vi "Format Wavename.vi"(8 "error in (no error)":errorcluster, 9 "Index":i32, 10 "Path":path, 11 "Name":string) -> (0 "error out":errorcluster, 3 "Formatted wavename":string)   [LabVIEW 2016, in "LV-Data.ITX.lvclass"]
uses:
  LV-Data.ITX.lvclass
  LV-Data/LV-Data.lvclass
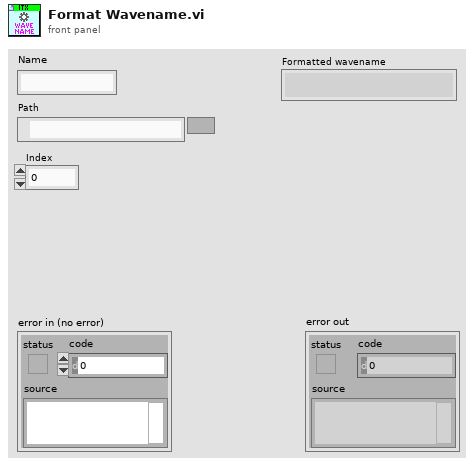
[diagram p1: front panel]
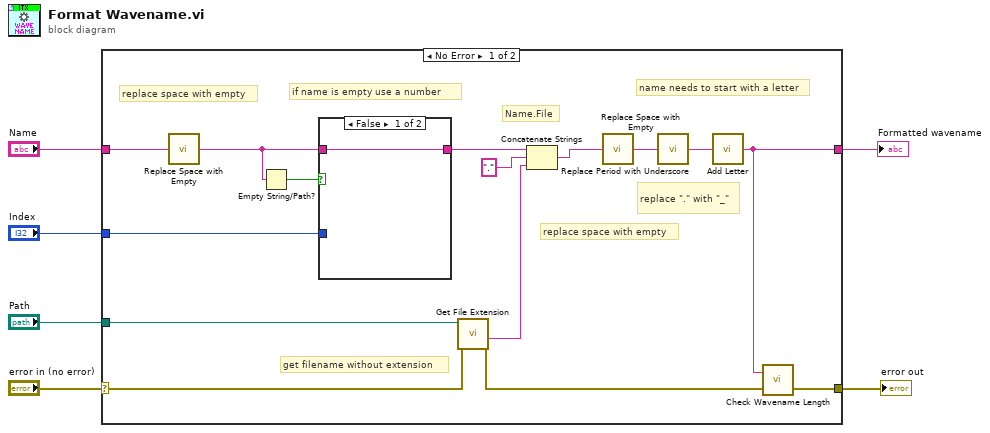
[diagram p0: block diagram]
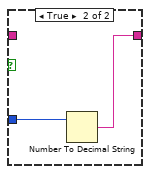
[diagram p2: hidden frame]
diagram:
  n1 = case shown="No Error" "error in (no error)" {
    selector: "error in (no error)" -> [w14 w26]
    tunnel: "Name" -> [w21 w25]
    tunnel: "Index" -> [w18 _]
    tunnel: "Path" -> [w16 _]
    tunnel: [w10 w25] -> w1
    tunnel: [w12 w26] -> w3
    frame No Error {
      # "replace space with empty"
      # "name needs to start with a letter"
      # "Name.File"
      # "if name is empty use a number"
      # "get filename without extension"
      # "replace \".\" with \"_\""
      # "replace space with empty"
      n2 = call "Replace Space with Empty.vi"("string"=w21) -> ("result string"=w13:string)
      n3 = Empty String/Path?(string/path=w13) -> (empty?=w17:bool)
      n4 = case shown="False" w17 {
        tunnel: w18 -> [_ w23]
        tunnel: [w22 w24] -> w19
        tunnel: w13 -> [w22 _]
        frame False {
        }
        frame True {
          n5 = Number To Decimal String(number=w23) -> (decimal integer string=w24:string)  [unwired: 1 out]
        }
      }
      n6 = call <vilib>:"Get File Extension.vi"("error in (no error)"=w14, "file"=w16) -> ("error out"=w9:errorcluster, "filename without extension"=w15:string)  [unwired: 5 in, 3 out]
      n7 = Concatenate Strings(w19, "." ("string"), w15) -> (w8:string)
      n8 = call "Replace Space with Empty.vi"("string"=w8) -> ("result string"=w7:string)
      n9 = call "Replace Period with Underscore.vi"("string"=w7) -> ("result string"=w11:string)
      n10 = call "Add Letter.vi"("string"=w11) -> ("result string"=w10:string)
      n11 = call "Check Wavename Length.vi"("error in (no error)"=w9, "Wavename"=w10) -> ("error out"=w12:errorcluster)  [unwired: 1 out]
    }
    frame Error {
    }
  }
  "Formatted wavename" <- w1
  "error out" <- w3
